vi "数据库.vi"() -> ()   [LabVIEW 2018]
uses:
  <vilib>/addons/database/Auxilliary.llb/DB Tools Column Info.ctl
  <vilib>/addons/database/Auxilliary.llb/DB Tools DataTypes.ctl
  <vilib>/addons/database/Connection.llb/DB Tools Open Connec (String).vi
  <vilib>/addons/database/NI_Database_API.lvlib
panel:
  in  "数组":dbl[][](array[numeric])
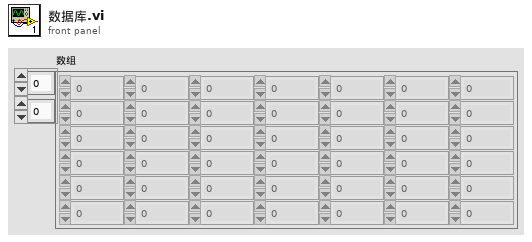
[diagram p1: front panel]
types:
  T1 = typedef "NI_Database_API.lvlib/DB Tools Column Info.ctl" = cluster{"column name":string, "data type":T2, "size":i32, "allow null?":bool}
  T2 = typedef "NI_Database_API.lvlib/DB Tools DataTypes.ctl" = enum16{"String", "Long (I32)", "Single (SGL)", "Double (DBL)", "Date/Time", "Binary"}
  T3 = typedef "NI_Database_API.lvlib/Conn ObjectReference.ctl" = refnum<k1>
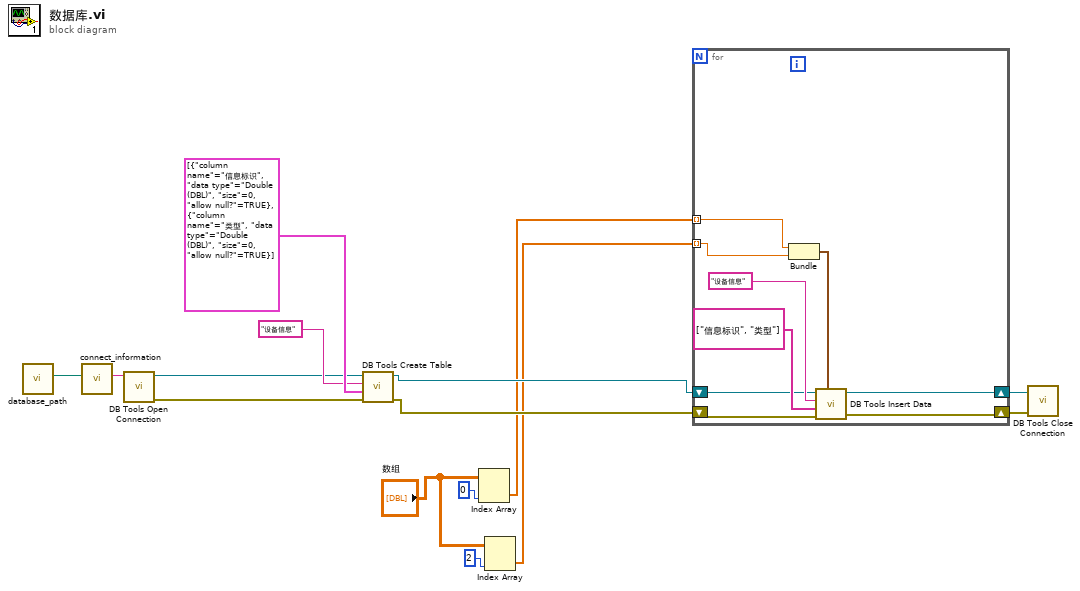
[diagram p0: block diagram]
diagram:
  n1 = call "database_path.vi"() -> ("database path"=w14:path)  [unwired: 11 in]
  n2 = call "connect_information.vi"("路径"=w14) -> ("connect info"=w15:string)  [unwired: 10 in]
  n3 = call-poly <vilib>:"DB Tools Open Connection.vi"("connection information"=w15) -> ("error out"=w10:errorcluster, "connection reference"=w11:T3)  [unwired: 7 in]
  n4 = call <vilib>:"DB Tools Create Table.vi"("error in (no error)"=w10, "column information"=T1[] [{"column name"="信息标识", "data type"=enum."Double (DBL)", "size"=0, "allow null?"=TRUE}, {"column name"="类型", "data type"=enum."Double (DBL)", "size"=0, "allow null?"=TRUE}], "table"="设备信息", "connection reference"=w11) -> ("error out"=w8:errorcluster, "connection reference out"=w9:T3)  [unwired: 4 in]
  n5 = Index Array(array="数组", index (col)=0 ("索引 (行)")) -> (element=w4:dbl[])  [unwired: 1 in]
  n6 = Index Array(array="数组", index (col)=2 ("索引 (行)")) -> (element=w3:dbl[])  [unwired: 1 in]
  n7 = for {
    shift-right: [w19] -> w7
    shift-left: w9 -> [w21]
    shift-right: [w18] -> w6
    shift-left: w8 -> [w20]
    tunnel: w4 -> [w16] mode=indexing
    tunnel: w3 -> [w17] mode=indexing
    n8 = Bundle("数值"=w16, "数值"=w17) -> (w24:cluster{"数值":dbl, "数值":dbl})  [unwired: 1 in]
    n9 = call <vilib>:"DB Tools Insert Data.vi"("data"=w24, "error in (no error)"=w20, "columns"=string[] ["信息标识", "类型"], "table"="设备信息", "connection reference"=w21) -> ("error out"=w18:errorcluster, "connection reference out"=w19:T3)  [unwired: 5 in]
  }
  n10 = call <vilib>:"DB Tools Close Connection.vi"("error in (no error)"=w6, "connection reference"=w7) -> ()  [unwired: 5 in, 1 out]
